vi "ExitLabVIEW_14.0.vi"() -> ()   [LabVIEW 2014]
panel:
  out "error out":errorcluster
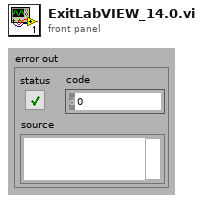
[diagram p1: front panel]
types:
  T1 = enum32{"Invalid", "Standard", "Closed", "Hidden", "Minimized", "Maximized"}
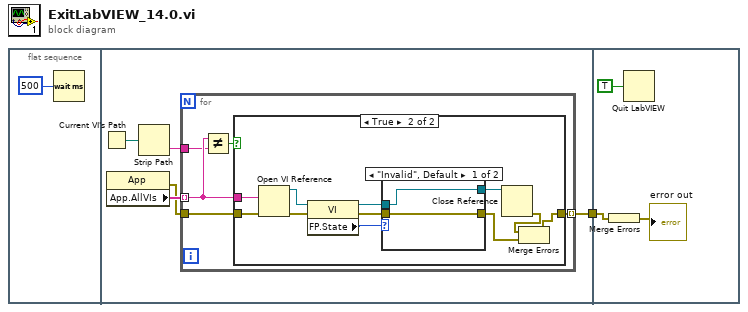
[diagram p0: block diagram]
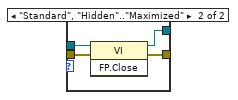
[diagram p3: hidden frame]
diagram:
  n1 = flat-sequence {
    tunnel: [w3] -> w1
    tunnel: w1 -> [w31]
    frame #0 {
      n2 = Wait (ms)(milliseconds to wait=u32 500) -> ()  [unwired: 1 out]
    }
    frame #1 {
      n3 = Current VI's Path() -> (path=w7:path)
      n4 = property class="App"() -> (error out=w4:errorcluster, "App.AllVIs"=w5:string[])  [unwired: 2 in, 1 out]
      n5 = Strip Path(path=w7) -> (name=w6:string)  [unwired: 1 out]
      n6 = for {
        tunnel: w5 -> [w11] mode=indexing
        tunnel: w6 -> [w10]
        tunnel: w4 -> [w9]
        tunnel: [w8] -> w3 mode=indexing
        n7 = Not Equal?(x=w11, y=w10) -> (x != y?=w12:bool)
        n8 = case shown="True" w12 {
          tunnel: w11 -> [_ w23]
          tunnel: [_ w13] -> w8
          tunnel: w9 -> [_ w16]
          frame False {
          }
          frame True {
            n9 = Open VI Reference(vi path=w23, error in (no error)=w16) -> (vi reference=w21:refnum<vi>, error out=w22:errorcluster)  [unwired: 4 in]
            n10 = property class="VI"(reference=w21, error in=w22) -> (reference out=w18:refnum<vi>, error out=w17:errorcluster, "FP.State"=w19:T1)
            n11 = case shown="\"Invalid\", Default" w19 {
              tunnel: w17 -> [w24 w29]
              tunnel: w18 -> [w25 w28]
              tunnel: [w25 w27] -> w20
              tunnel: [w24 w26] -> w14
              frame "Invalid", Default {
              }
              frame "Standard", "Hidden".."Maximized" {
                n12 = invoke class="VI" method="FP.Close"(reference=w28, error in=w29) -> (reference out=w27:refnum<vi>, error out=w26:errorcluster)  [unwired: 1 in, 1 out]
              }
            }
            n13 = Close Reference(reference=w20) -> (error out=w15:errorcluster)  [unwired: 1 in]
            n14 = Merge Errors(w15, w14) -> (w13:errorcluster)
          }
        }
      }
    }
    frame #2 {
      n15 = Merge Errors(w31) -> (→"error out":errorcluster)
      n16 = Quit LabVIEW(quit? (T)=TRUE) -> ()
    }
  }
